vi "Persistence_Main.vi"() -> ()   [LabVIEW 2016]
uses:
  Data Hyway TD.ctl
  Que Attributes TD.ctl
  Que enum td.ctl
panel:
  in  "Log":bool
  in  "PP_value":dbl
  in  "PP_HOME":bool
  in  "PP_STOP":bool
  in  "PP_START":bool
  in  "Connect":bool
  in  "Exit":bool
  # "Pitchpack"
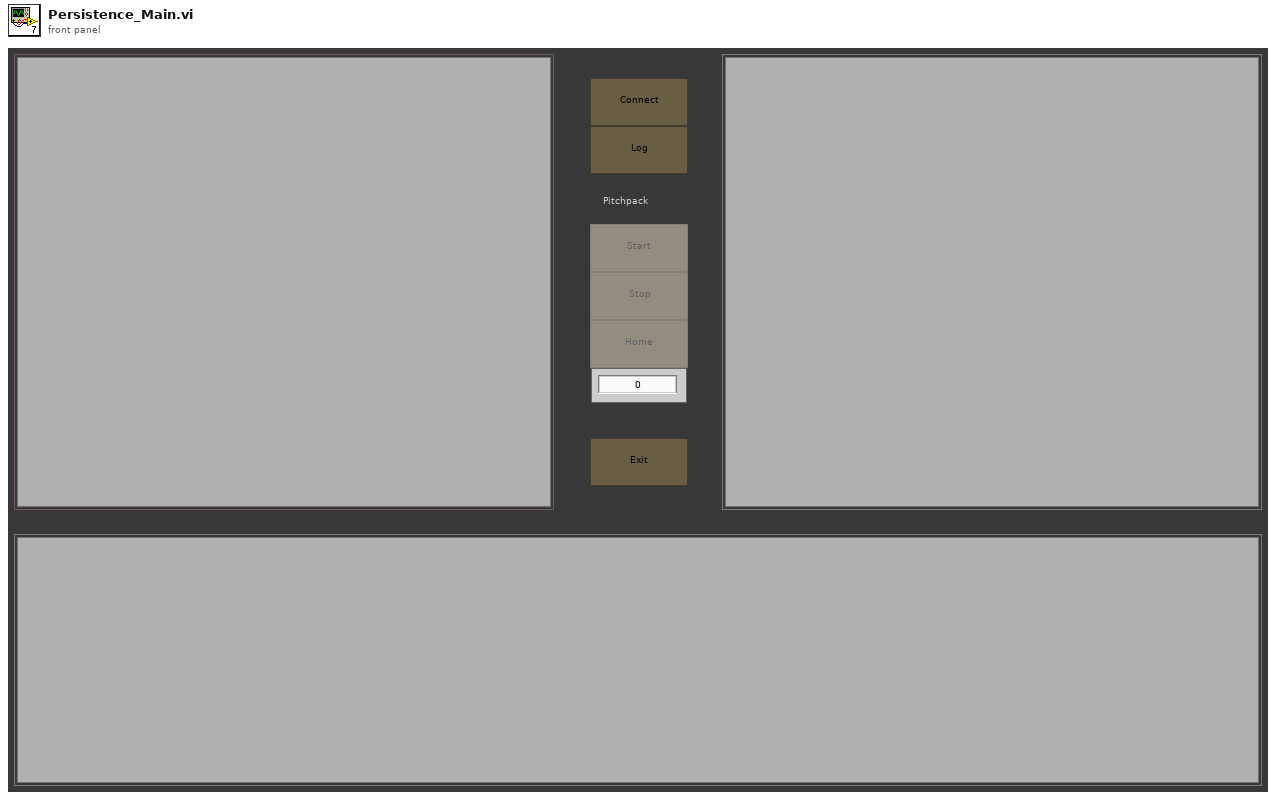
[diagram p1: front panel]
types:
  T1 = typedef "Data Hyway TD.ctl" = cluster{"PP_value":dbl, "String":string, "Boolean":bool}
  T2 = typedef "Que Cluster TD.ctl" = cluster{"Main":refnum<queue>, "ZMQ_SUB":refnum<queue>, "External":refnum<queue>, "Vibration":refnum<queue>, "ZMQ_REQ":refnum<queue>}
  T3 = typedef "Que Attributes TD.ctl" = cluster{"Que States":T4, "String":string, "Boolean":bool, "Double":dbl, "U16":u16}
  T4 = typedef "Que enum td.ctl" = enum16{"Stop", "Start", "Update D_HW", "Initialize", "Exit", "Read", "Write", "Plot", "Log", "Stop Log", "Start Log", "Wait"}
  T5 = typedef "Que Atributes TD.ctl" = cluster{"Que States":T4, "String":string, "Boolean":bool, "Double":dbl, "U16":u16}
  T6 = enum8{"Enabled", "Disabled", "Disabled and Grayed Out"}
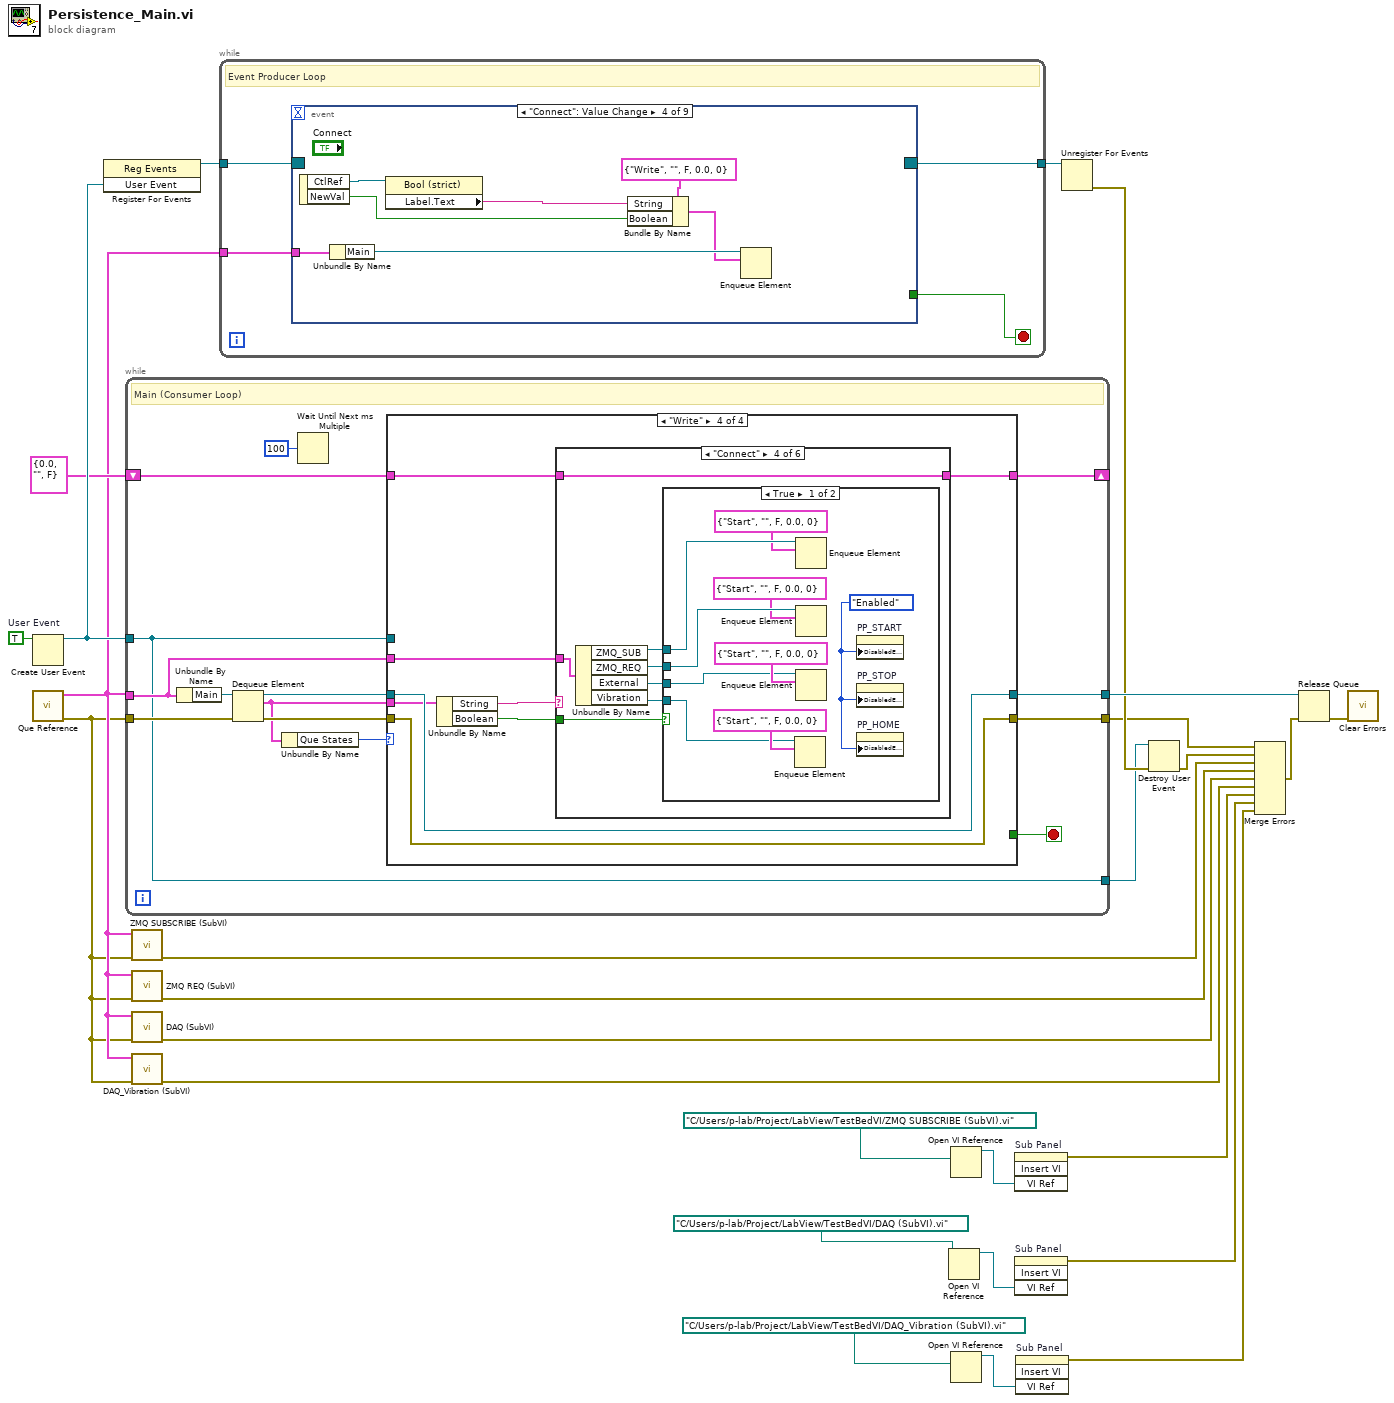
[diagram p0: block diagram]
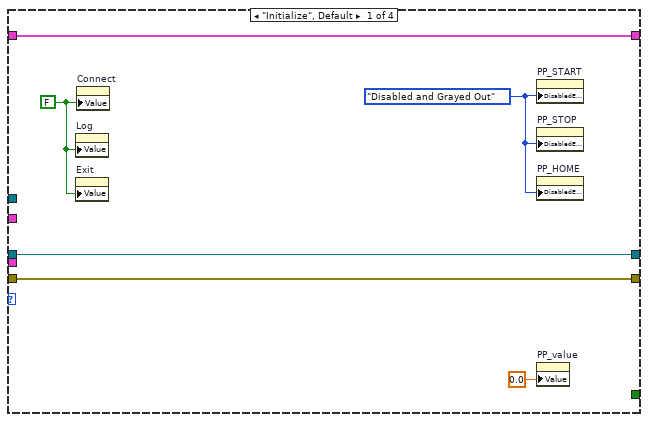
[diagram p2: hidden frame]
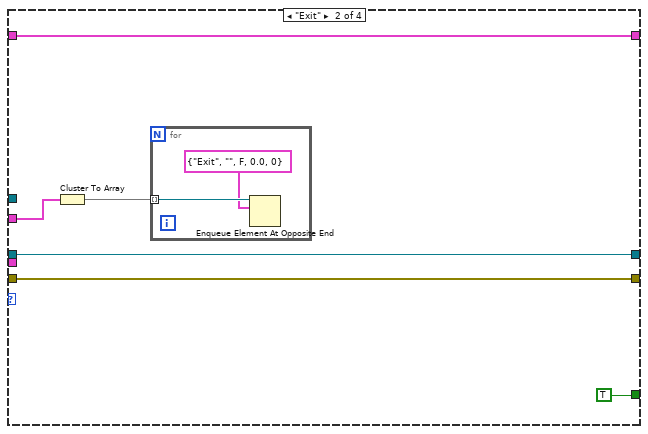
[diagram p3: hidden frame]
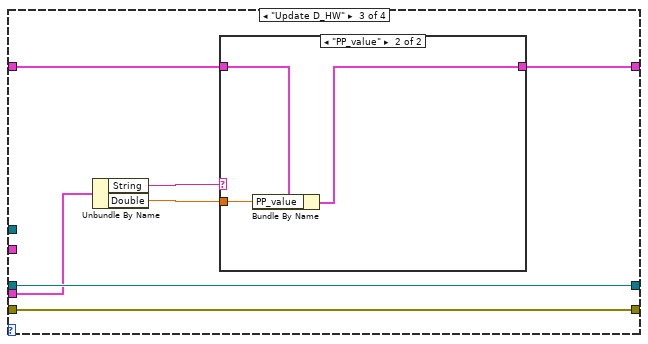
[diagram p4: hidden frame]
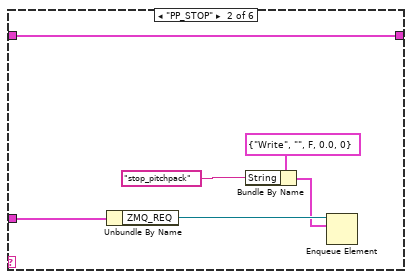
[diagram p7: hidden frame]
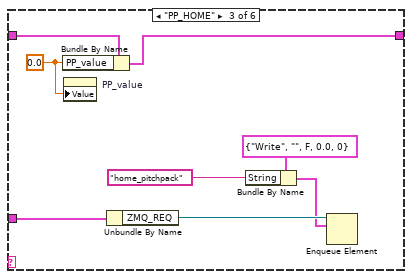
[diagram p8: hidden frame]
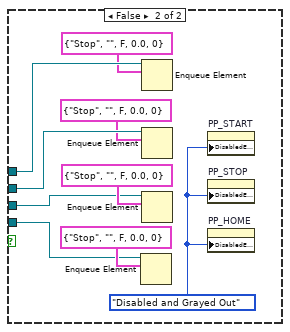
[diagram p9: hidden frame]
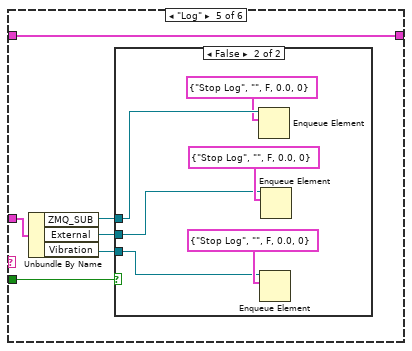
[diagram p10: hidden frame]
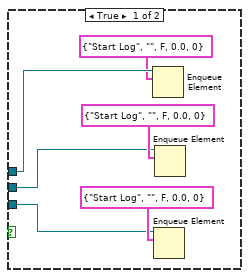
[diagram p11: hidden frame]
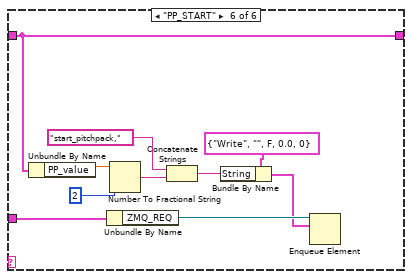
[diagram p12: hidden frame]
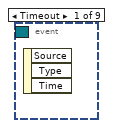
[diagram p13: hidden frame]
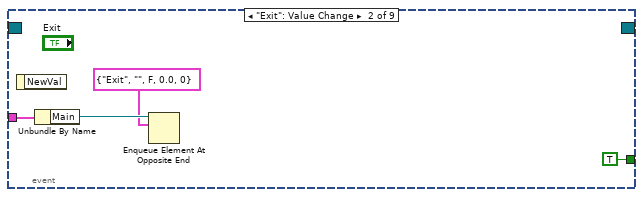
[diagram p14: hidden frame]
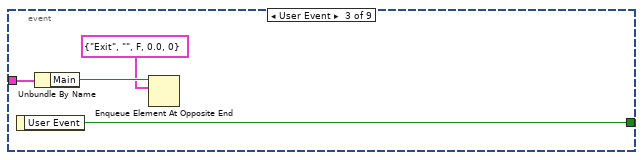
[diagram p15: hidden frame]
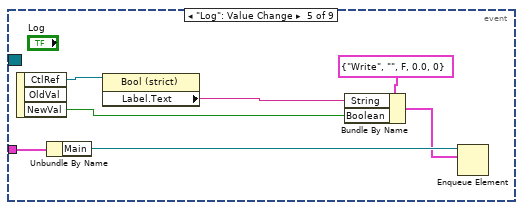
[diagram p16: hidden frame]
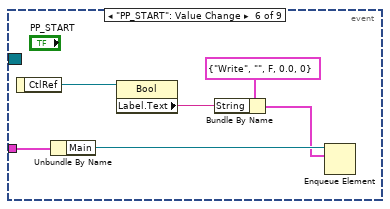
[diagram p17: hidden frame]
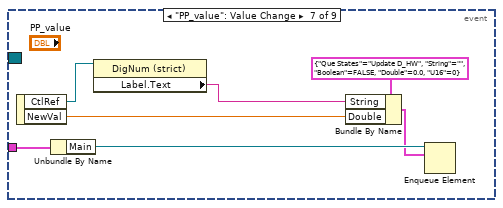
[diagram p18: hidden frame]
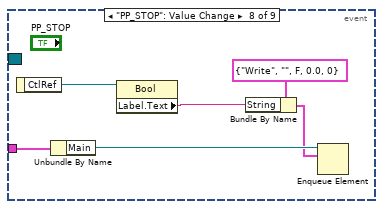
[diagram p19: hidden frame]
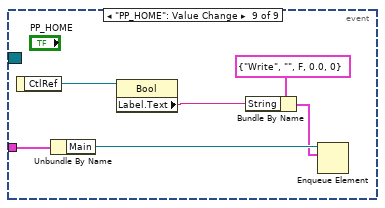
[diagram p20: hidden frame]
diagram:
  w26 = TRUE  # User Event
  n1 = Create User Event(user event datatype=w26) -> (user event=w25:refnum<user-event>)  [unwired: 1 in, 1 out]
  n2 = call "Que Reference.vi"() -> ("error out"=w7:errorcluster, "output cluster"=w8:T2)  [unwired: 10 in]
  n3 = register-events(w25) -> (reference out=w24:refnum<event-registration>)  [unwired: 2 in, 1 out]
  n4 = while {
    tunnel: w7 -> [w40]
    tunnel: w8 -> [w34]
    tunnel: [w37] -> w27
    tunnel: [w36] -> w18
    tunnel: w25 -> [w31]
    shift-right: [w32] -> _
    shift-left: T1 {"PP_value"=0.0, "String"="", "Boolean"=FALSE} ("Data Hyway") -> [w33]
    tunnel: [w31] -> w20
    stop <- w29 stop-if-true
    # "Main (Consumer Loop)"
    n5 = Unbundle By Name(w34) -> ("Main"=w41:refnum<queue>)
    n6 = Dequeue Element(queue=w41, error in (no error)=w40) -> (queue out=w39:refnum<queue>, element=w28:T5, error out=w38:errorcluster)  [unwired: 1 in, 1 out]
    n7 = Unbundle By Name(w28) -> ("Que States"=w35:T4)
    n8 = Wait Until Next ms Multiple(millisecond multiple=u32 100) -> ()  [unwired: 1 out]
    n9 = case shown="\"Write\"" w35 {
      tunnel: w39 -> [w47 w53 w62 w73]
      tunnel: w38 -> [w46 w52 w59 w68]
      tunnel: [w47 w53 w62 w73] -> w37
      tunnel: [w46 w52 w59 w68] -> w36
      tunnel: w34 -> [_ w50 _ w74]
      tunnel: w31 -> [_ _ _ _]
      tunnel: w33 -> [w45 w51 w61 w72]
      tunnel: [w45 w51 w60 w71] -> w32
      tunnel: [_ TRUE _ _] -> w29
      tunnel: w28 -> [_ _ w58 w70]
      frame "Initialize", Default {
        w42 = FALSE ("Connect")
        w44 = T6."Disabled and Grayed Out" ("Disabled")
        n10 = property on="Log" class="Bool (strict)"("Value"=w42) -> ()  [unwired: 2 in, 2 out]
        n11 = property on="Exit" class="Bool (strict)"("Value"=w42) -> ()  [unwired: 2 in, 2 out]
        n12 = property on="Connect" class="Bool (strict)"("Value"=w42) -> ()  [unwired: 2 in, 2 out]
        n13 = property on="PP_START" class="Bool"("DisabledEnum"=w44) -> ()  [unwired: 2 in, 2 out]
        n14 = property on="PP_STOP" class="Bool"("DisabledEnum"=w44) -> ()  [unwired: 2 in, 2 out]
        n15 = property on="PP_HOME" class="Bool"("DisabledEnum"=w44) -> ()  [unwired: 2 in, 2 out]
        n16 = property on="PP_value" class="DigNum (strict)"("Value"=0.0 ("PP_value")) -> ()  [unwired: 2 in, 2 out]
      }
      frame "Exit" {
        n17 = Cluster To Array(cluster=w50) -> (array=w49:refnum<queue>[])
        n18 = for {
          tunnel: w49 -> [w55] mode=indexing
          n19 = Enqueue Element At Opposite End(queue=w55, element=T3 {"Que States"=enum."Exit", "String"="", "Boolean"=FALSE, "Double"=0.0, "U16"=0}) -> ()  [unwired: 2 in, 3 out]
        }
      }
      frame "Update D_HW" {
        n20 = Unbundle By Name(w58) -> ("String"=w57:string, "Double"=w56:dbl)
        n21 = case shown="\"PP_value\"" w57 {
          tunnel: w61 -> [w63 w66]
          tunnel: [w63 w65] -> w60
          tunnel: w56 -> [_ w64]
          frame "False", Default {
          }
          frame "PP_value" {
            n22 = Bundle By Name(cluster=w66, "PP_value"=w64) -> (w65:T1)
          }
        }
      }
      frame "Write" {
        n23 = Unbundle By Name(w70) -> ("String"=w69:string, "Boolean"=w67:bool)
        n24 = case shown="\"Connect\"" w69 {
          tunnel: w74 -> [_ w81 w89 w95 w119 w142]
          tunnel: w72 -> [w75 w78 w86 w96 w120 w137]
          tunnel: [w75 w78 w85 w96 w120 w137] -> w71
          tunnel: w67 -> [_ _ _ w92 w117 _]
          frame "False", Default {
          }
          frame "PP_STOP" {
            n25 = Unbundle By Name(w81) -> ("ZMQ_REQ"=w80:refnum<queue>)
            n26 = Bundle By Name(cluster=T3 {"Que States"=enum."Write", "String"="", "Boolean"=FALSE, "Double"=0.0, "U16"=0} ("element"), "String"="stop_pitchpack") -> (w76:T3)
            n27 = Enqueue Element(queue=w80, element=w76) -> ()  [unwired: 2 in, 3 out]
          }
          frame "PP_HOME" {
            w82 = 0.0 ("PP_value")
            n28 = Bundle By Name(cluster=w86, "PP_value"=w82) -> (w85:T1)
            n29 = property on="PP_value" class="DigNum (strict)"("Value"=w82) -> ()  [unwired: 2 in, 2 out]
            n30 = Unbundle By Name(w89) -> ("ZMQ_REQ"=w88:refnum<queue>)
            n31 = Bundle By Name(cluster=T3 {"Que States"=enum."Write", "String"="", "Boolean"=FALSE, "Double"=0.0, "U16"=0} ("element"), "String"="home_pitchpack") -> (w83:T3)
            n32 = Enqueue Element(queue=w88, element=w83) -> ()  [unwired: 2 in, 3 out]
          }
          frame "Connect" {
            n33 = Unbundle By Name(w95) -> ("ZMQ_SUB"=w94:refnum<queue>, "ZMQ_REQ"=w93:refnum<queue>, "External"=w91:refnum<queue>, "Vibration"=w90:refnum<queue>)
            n34 = case shown="True" w92 {
              tunnel: w94 -> [w105 w114]
              tunnel: w93 -> [w104 w113]
              tunnel: w91 -> [w99 w108]
              tunnel: w90 -> [w97 w106]
              frame True {
                w103 = T6."Enabled" ("Disabled")
                n35 = Enqueue Element(queue=w97, element=T3 {"Que States"=enum."Start", "String"="", "Boolean"=FALSE, "Double"=0.0, "U16"=0}) -> ()  [unwired: 2 in, 3 out]
                n36 = Enqueue Element(queue=w105, element=T3 {"Que States"=enum."Start", "String"="", "Boolean"=FALSE, "Double"=0.0, "U16"=0}) -> ()  [unwired: 2 in, 3 out]
                n37 = Enqueue Element(queue=w104, element=T3 {"Que States"=enum."Start", "String"="", "Boolean"=FALSE, "Double"=0.0, "U16"=0}) -> ()  [unwired: 2 in, 3 out]
                n38 = Enqueue Element(queue=w99, element=T3 {"Que States"=enum."Start", "String"="", "Boolean"=FALSE, "Double"=0.0, "U16"=0}) -> ()  [unwired: 2 in, 3 out]
                n39 = property on="PP_START" class="Bool"("DisabledEnum"=w103) -> ()  [unwired: 2 in, 2 out]
                n40 = property on="PP_STOP" class="Bool"("DisabledEnum"=w103) -> ()  [unwired: 2 in, 2 out]
                n41 = property on="PP_HOME" class="Bool"("DisabledEnum"=w103) -> ()  [unwired: 2 in, 2 out]
              }
              frame False {
                w112 = T6."Disabled and Grayed Out" ("Disabled")
                n42 = Enqueue Element(queue=w106, element=T3 {"Que States"=enum."Stop", "String"="", "Boolean"=FALSE, "Double"=0.0, "U16"=0}) -> ()  [unwired: 2 in, 3 out]
                n43 = Enqueue Element(queue=w114, element=T3 {"Que States"=enum."Stop", "String"="", "Boolean"=FALSE, "Double"=0.0, "U16"=0}) -> ()  [unwired: 2 in, 3 out]
                n44 = Enqueue Element(queue=w113, element=T3 {"Que States"=enum."Stop", "String"="", "Boolean"=FALSE, "Double"=0.0, "U16"=0}) -> ()  [unwired: 2 in, 3 out]
                n45 = Enqueue Element(queue=w108, element=T3 {"Que States"=enum."Stop", "String"="", "Boolean"=FALSE, "Double"=0.0, "U16"=0}) -> ()  [unwired: 2 in, 3 out]
                n46 = property on="PP_START" class="Bool"("DisabledEnum"=w112) -> ()  [unwired: 2 in, 2 out]
                n47 = property on="PP_STOP" class="Bool"("DisabledEnum"=w112) -> ()  [unwired: 2 in, 2 out]
                n48 = property on="PP_HOME" class="Bool"("DisabledEnum"=w112) -> ()  [unwired: 2 in, 2 out]
              }
            }
          }
          frame "Log" {
            n49 = Unbundle By Name(w119) -> ("ZMQ_SUB"=w118:refnum<queue>, "External"=w116:refnum<queue>, "Vibration"=w115:refnum<queue>)
            n50 = case shown="False" w117 {
              tunnel: w118 -> [w126 w132]
              tunnel: w116 -> [w123 w129]
              tunnel: w115 -> [w121 w127]
              frame True {
                n51 = Enqueue Element(queue=w126, element=T3 {"Que States"=enum."Start Log", "String"="", "Boolean"=FALSE, "Double"=0.0, "U16"=0}) -> ()  [unwired: 2 in, 3 out]
                n52 = Enqueue Element(queue=w121, element=T3 {"Que States"=enum."Start Log", "String"="", "Boolean"=FALSE, "Double"=0.0, "U16"=0}) -> ()  [unwired: 2 in, 3 out]
                n53 = Enqueue Element(queue=w123, element=T3 {"Que States"=enum."Start Log", "String"="", "Boolean"=FALSE, "Double"=0.0, "U16"=0}) -> ()  [unwired: 2 in, 3 out]
              }
              frame False {
                n54 = Enqueue Element(queue=w132, element=T3 {"Que States"=enum."Stop Log", "String"="", "Boolean"=FALSE, "Double"=0.0, "U16"=0}) -> ()  [unwired: 2 in, 3 out]
                n55 = Enqueue Element(queue=w127, element=T3 {"Que States"=enum."Stop Log", "String"="", "Boolean"=FALSE, "Double"=0.0, "U16"=0}) -> ()  [unwired: 2 in, 3 out]
                n56 = Enqueue Element(queue=w129, element=T3 {"Que States"=enum."Stop Log", "String"="", "Boolean"=FALSE, "Double"=0.0, "U16"=0}) -> ()  [unwired: 2 in, 3 out]
              }
            }
          }
          frame "PP_START" {
            n57 = Unbundle By Name(w137) -> ("PP_value"=w140:dbl)
            n58 = Unbundle By Name(w142) -> ("ZMQ_REQ"=w141:refnum<queue>)
            n59 = Number To Fractional String(number=w140, precision (6)=i16 2) -> (F-format string=w138:string)  [unwired: 2 in]
            n60 = Concatenate Strings("start_pitchpack,", w138) -> (w135:string)
            n61 = Bundle By Name(cluster=T3 {"Que States"=enum."Write", "String"="", "Boolean"=FALSE, "Double"=0.0, "U16"=0} ("element"), "String"=w135) -> (w134:T3)
            n62 = Enqueue Element(queue=w141, element=w134) -> ()  [unwired: 2 in, 3 out]
          }
        }
      }
    }
  }
  n63 = call "ZMQ SUBSCRIBE (SubVI).vi"("error in (no error)"=w7, "output cluster"=w8) -> ("error out"=w11:errorcluster)  [unwired: 9 in]
  n64 = call "ZMQ REQ (SubVI).vi"("error in (no error)"=w7, "output cluster"=w8) -> ("error out"=w10:errorcluster)  [unwired: 9 in]
  n65 = call "DAQ (SubVI).vi"("error in (no error)"=w7, "output cluster"=w8) -> ("error out"=w9:errorcluster)  [unwired: 9 in]
  n66 = call "DAQ_Vibration (SubVI).vi"("error in (no error)"=w7, "output cluster"=w8) -> ("error out"=w1:errorcluster)  [unwired: 9 in]
  n67 = while {
    tunnel: w8 -> [w146]
    tunnel: w24 -> [w144]
    tunnel: [w143] -> w22
    stop <- w145 stop-if-true
    # "Event Producer Loop"
    n68 = event shown="[3] \"Connect\": Value Change" {
      selector: w144 -> [_ _ _ _ _ _ _ _ _]
      dyn-events: [_ _ _ _ _ _ _ _ _] -> w143
      timeout: _ -> [_ _ _ _ _ _ _ _ _]
      tunnel: w146 -> [_ w150 w154 w161 w168 w174 w181 w187 w193]
      tunnel: [_ TRUE ("User Event") w152 _ _ _ _ _ _] -> w145
      event Timeout {
        n69 = event-data() -> ()  [unwired: 1 in, 3 out]
      }
      event "Exit": Value Change {
        n70 = event-data() -> ()  [unwired: 1 in, 1 out]
        n71 = Unbundle By Name(w150) -> ("Main"=w149:refnum<queue>)
        n72 = Enqueue Element At Opposite End(queue=w149, element=T3 {"Que States"=enum."Exit", "String"="", "Boolean"=FALSE, "Double"=0.0, "U16"=0}) -> ()  [unwired: 2 in, 3 out]
      }
      event User Event {
        n73 = event-data() -> ("User Event"=w152:bool)  [unwired: 1 in]
        n74 = Unbundle By Name(w154) -> ("Main"=w153:refnum<queue>)
        n75 = Enqueue Element At Opposite End(queue=w153, element=T3 {"Que States"=enum."Exit", "String"="", "Boolean"=FALSE, "Double"=0.0, "U16"=0}) -> ()  [unwired: 2 in, 3 out]
      }
      event "Connect": Value Change {
        n76 = event-data() -> ("CtlRef"=w159:refnum<vi>, "NewVal"=w156:bool)  [unwired: 1 in]
        n77 = Unbundle By Name(w161) -> ("Main"=w160:refnum<queue>)
        n78 = property class="Bool (strict)"(reference=w159) -> ("Label.Text"=w157:string)  [unwired: 1 in, 2 out]
        n79 = Bundle By Name(cluster=T3 {"Que States"=enum."Write", "String"="", "Boolean"=FALSE, "Double"=0.0, "U16"=0} ("element"), "String"=w157, "Boolean"=w156) -> (w155:T3)
        n80 = Enqueue Element(queue=w160, element=w155) -> ()  [unwired: 2 in, 3 out]
      }
      event "Log": Value Change {
        n81 = event-data() -> ("CtlRef"=w166:refnum<vi>, "NewVal"=w162:bool)  [unwired: 1 in, 1 out]
        n82 = Unbundle By Name(w168) -> ("Main"=w167:refnum<queue>)
        n83 = property class="Bool (strict)"(reference=w166) -> ("Label.Text"=w164:string)  [unwired: 1 in, 2 out]
        n84 = Bundle By Name(cluster=T3 {"Que States"=enum."Write", "String"="", "Boolean"=FALSE, "Double"=0.0, "U16"=0} ("element"), "String"=w164, "Boolean"=w162) -> (w163:T3)
        n85 = Enqueue Element(queue=w167, element=w163) -> ()  [unwired: 2 in, 3 out]
      }
      event "PP_START": Value Change {
        n86 = event-data() -> ("CtlRef"=w172:refnum<vi>)  [unwired: 1 in]
        n87 = Unbundle By Name(w174) -> ("Main"=w173:refnum<queue>)
        n88 = property class="Bool"(reference=w172) -> ("Label.Text"=w171:string)  [unwired: 1 in, 2 out]
        n89 = Bundle By Name(cluster=T3 {"Que States"=enum."Write", "String"="", "Boolean"=FALSE, "Double"=0.0, "U16"=0} ("element"), "String"=w171) -> (w169:T3)
        n90 = Enqueue Element(queue=w173, element=w169) -> ()  [unwired: 2 in, 3 out]
      }
      event "PP_value": Value Change {
        n91 = event-data() -> ("CtlRef"=w179:refnum<vi>, "NewVal"=w176:dbl)  [unwired: 1 in]
        n92 = Unbundle By Name(w181) -> ("Main"=w180:refnum<queue>)
        n93 = property class="DigNum (strict)"(reference=w179) -> ("Label.Text"=w177:string)  [unwired: 1 in, 2 out]
        n94 = Bundle By Name(cluster=T3 {"Que States"=enum."Update D_HW", "String"="", "Boolean"=FALSE, "Double"=0.0, "U16"=0} ("element"), "String"=w177, "Double"=w176) -> (w175:T3)
        n95 = Enqueue Element(queue=w180, element=w175) -> ()  [unwired: 2 in, 3 out]
      }
      event "PP_STOP": Value Change {
        n96 = event-data() -> ("CtlRef"=w185:refnum<vi>)  [unwired: 1 in]
        n97 = Unbundle By Name(w187) -> ("Main"=w186:refnum<queue>)
        n98 = property class="Bool"(reference=w185) -> ("Label.Text"=w183:string)  [unwired: 1 in, 2 out]
        n99 = Bundle By Name(cluster=T3 {"Que States"=enum."Write", "String"="", "Boolean"=FALSE, "Double"=0.0, "U16"=0} ("element"), "String"=w183) -> (w182:T3)
        n100 = Enqueue Element(queue=w186, element=w182) -> ()  [unwired: 2 in, 3 out]
      }
      event "PP_HOME": Value Change {
        n101 = event-data() -> ("CtlRef"=w191:refnum<vi>)  [unwired: 1 in]
        n102 = Unbundle By Name(w193) -> ("Main"=w192:refnum<queue>)
        n103 = property class="Bool"(reference=w191) -> ("Label.Text"=w189:string)  [unwired: 1 in, 2 out]
        n104 = Bundle By Name(cluster=T3 {"Que States"=enum."Write", "String"="", "Boolean"=FALSE, "Double"=0.0, "U16"=0} ("element"), "String"=w189) -> (w188:T3)
        n105 = Enqueue Element(queue=w192, element=w188) -> ()  [unwired: 2 in, 3 out]
      }
    }
  }
  n106 = Open VI Reference(vi path=path "C:/Users/p-lab/Project/LabView/TestBedVI/DAQ (SubVI).vi") -> (vi reference=w13:refnum<vi>)  [unwired: 5 in, 1 out]
  n107 = Open VI Reference(vi path=path "C:/Users/p-lab/Project/LabView/TestBedVI/ZMQ SUBSCRIBE (SubVI).vi") -> (vi reference=w16:refnum<vi>)  [unwired: 5 in, 1 out]
  n108 = Open VI Reference(vi path=path "C:/Users/p-lab/Project/LabView/TestBedVI/DAQ_Vibration (SubVI).vi") -> (vi reference=w6:refnum<vi>)  [unwired: 5 in, 1 out]
  n109 = invoke on="Sub Panel" class="SubPnl" method="Insert VI"("VI Ref"=w16) -> (error out=w2:errorcluster)  [unwired: 3 in, 3 out]
  n110 = invoke on="Sub Panel" class="SubPnl" method="Insert VI"("VI Ref"=w13) -> (error out=w3:errorcluster)  [unwired: 3 in, 3 out]
  n111 = invoke on="Sub Panel" class="SubPnl" method="Insert VI"("VI Ref"=w6) -> (error out=w4:errorcluster)  [unwired: 3 in, 3 out]
  n112 = Unregister For Events(event registration refnum=w22) -> (error out=w21:errorcluster)  [unwired: 1 in]
  n113 = Destroy User Event(user event=w20, error in=w21) -> (error out=w19:errorcluster)
  n114 = Merge Errors(w18, w19, w11, w10, w9, w1, w2, w3, w4) -> (w17:errorcluster)
  n115 = Release Queue(queue=w27, error in (no error)=w17) -> (error out=w14:errorcluster)  [unwired: 1 in, 2 out]
  n116 = call <vilib>:"Clear Errors.vi"("error in (no error)"=w14) -> ()  [unwired: 5 in, 2 out]
